vi "PQ-12 quick release (SubVI).vi"(1 "error in (no error)":errorcluster, 2 "output cluster":T26 {"A/SPI - LiDAR"."SPI Configuration"."Frame Length" min=1 max=16}, 3 "Extend / Retract [F/T]":bool) -> (0 "error out":errorcluster)   [LabVIEW 2018]
uses:
  <vilib>/myRIO/Instrument Drivers/Onboard IO/DIO/typedefs/DIO Reference.ctl
  <vilib>/myRIO/Common/Instrument Driver Framework/Utilities/typedefs/myRIO Generic Hardware Reference.ctl
  <vilib>/myRIO/Common/Instrument Driver Framework/Utilities/typedefs/Hardware Version Enum.ctl
  <vilib>/myRIO/Common/Instrument Driver Framework/Utilities/typedefs/myRIO v1.0 Reference.ctl
  <vilib>/myRIO/Common/Instrument Driver Framework/Utilities/typedefs/Generic FPGA Reference.ctl
  <vilib>/myRIO/Common/Instrument Driver Framework/myRIO v1.0/DIO/typedefs/DIO Channels List.ctl
  <vilib>/myRIO/Common/Instrument Driver Framework/myRIO v1.0/DIO/typedefs/DIO Channels Enum.ctl
  <vilib>/myRIO/Instrument Drivers/Onboard IO/PWM/typedefs/PWM Reference.ctl
  <vilib>/myRIO/Common/Instrument Driver Framework/myRIO v1.0/PWM/typedefs/PWM Channels Enum.ctl
  <vilib>/myRIO/Instrument Drivers/Onboard IO/PWM/typedefs/PWM Configuration.ctl
  <vilib>/myRIO/Instrument Drivers/Onboard Devices/Accelerometer/typedefs/Accelerometer Reference.ctl
  <vilib>/myRIO/Common/Instrument Driver Framework/myRIO v1.0/Accelerometer/typedefs/Accelerometer Channels List.ctl
  <vilib>/myRIO/Common/Instrument Driver Framework/myRIO v1.0/Accelerometer/typedefs/Accelerometer Channels Enum.ctl
  <vilib>/myRIO/Instrument Drivers/Onboard IO/AI/typedefs/AI Reference.ctl
  <vilib>/myRIO/Common/Instrument Driver Framework/myRIO v1.0/AI/typedefs/AI Channels List.ctl
  <vilib>/myRIO/Common/Instrument Driver Framework/myRIO v1.0/AI/typedefs/AI Channels Enum.ctl
  <vilib>/myRIO/Common/Instrument Driver Framework/Utilities/typedefs/Analog Scaling Constants List.ctl
  <vilib>/myRIO/Common/Instrument Driver Framework/Utilities/typedefs/Analog Scaling Constants.ctl
  <vilib>/myRIO/Instrument Drivers/Onboard IO/SPI/typedefs/SPI Reference.ctl
  <vilib>/myRIO/Common/Instrument Driver Framework/myRIO v1.0/SPI/typedefs/SPI Channels Enum.ctl
  <vilib>/myRIO/Instrument Drivers/Onboard IO/SPI/typedefs/SPI Configuration.ctl
  <vilib>/myRIO/Common/Instrument Driver Framework/myRIO v1.0/SPI/typedefs/SPI Clock Phase.ctl
  <vilib>/myRIO/Common/Instrument Driver Framework/myRIO v1.0/SPI/typedefs/SPI Clock Polarity.ctl
  <vilib>/myRIO/Common/Instrument Driver Framework/myRIO v1.0/SPI/typedefs/SPI Data Direction.ctl
  <vilib>/myRIO/Common/Instrument Driver Framework/myRIO v1.0/SPI/typedefs/SPI Frame Length.ctl
  <vilib>/Utility/error.llb/Error Cluster From Error Code.vi
  <vilib>/myRIO/Common/Instrument Driver Framework/myRIO v1.0/AI/vis/myRIO v1.0 Read AI.vi
  <vilib>/myRIO/Common/Instrument Driver Framework/myRIO v1.0/DIO/vis/myRIO v1.0 Write DIO.vi
  <vilib>/myRIO/Instrument Drivers/Onboard IO/AI/AI.lvlib
  <vilib>/myRIO/Instrument Drivers/Onboard IO/DIO/DIO.lvlib
  <vilib>/myRIO/Instrument Drivers/Onboard IO/SPI/SPI.lvlib
  <vilib>/myRIO/Instrument Drivers/Onboard Devices/Accelerometer/Accelerometer.lvlib
  <vilib>/myRIO/Instrument Drivers/Onboard IO/PWM/PWM.lvlib
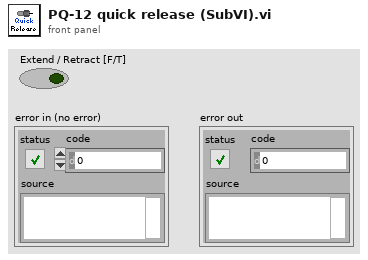
[diagram p1: front panel]
types:
  T1 = typedef "DIO.lvlib/DIO Reference.ctl" = cluster{"myRIO Reference":T2, "DIO Channels List":T6}
  T2 = typedef "myRIO Generic Hardware Reference.ctl" = cluster{"myRIO Model":T3, "myRIO Hardware Reference":T4}
  T3 = typedef "Hardware Version Enum.ctl" = enum16{"Unknown", "myRIO-1900", "myRIO-1950", "roboRIO", "NI ELVIS RIO CM", "ELVIS III"}
  T4 = typedef "myRIO v1.0 Reference.ctl" = cluster{"Generic FPGA Reference":T5, "Allow multiple opens":bool}
  T5 = typedef "Generic FPGA Reference.ctl" = refnum<k20>
  T6 = typedef "DIO Channels List.ctl" = T7[]
  T7 = typedef "DIO Channels Enum.ctl" = enum16{"Not Connected", "C/DIO0", "C/DIO1", "C/DIO2", "C/DIO3", "C/DIO4", "C/DIO5", "C/DIO6", "C/DIO7", "A/DIO0", "A/DIO1", "A/DIO2", "A/DIO3", "A/DIO4", "A/DIO5", "A/DIO6", "A/DIO7", "A/DIO8", "A/DIO9", "A/DIO10", "A/DIO11", "A/DIO12", "A/DIO13", "A/DIO14", "A/DIO15", "A/DIO16", "A/DIO17", "A/DIO18", "A/DIO19", "B/DIO0", "B/DIO1", "B/DIO2", "B/DIO3", "B/DIO4", "B/DIO5", "B/DIO6", "B/DIO7", "B/DIO8", "B/DIO9", "B/DIO10", "B/DIO11", "B/DIO12", "B/DIO13", "B/DIO14", "B/DIO15", "B/DIO16", "B/DIO17", "B/DIO18", "B/DIO19", "LED0", "LED1", "LED2", "LED3", "Button0", "DIO/DIO0", "DIO/DIO1", "DIO/DIO2", "DIO/DIO3", "DIO/DIO4", "DIO/DIO5", "DIO/DIO6", "DIO/DIO7", "DIO/DIO8", "DIO/DIO9", "SPI/CS0", "SPI/CS1", "SPI/CS2", "SPI/CS3", "LED RADIO (Green)", "LED RADIO (Red)", "LED COMM (Green)", "LED COMM (Red)", "LED MODE (Green)", "LED MODE (Red)"}
  T8 = typedef "PWM.lvlib/PWM Reference.ctl" = cluster{"myRIO Reference":T2, "PWM Channels Enum":T9, "PWM Configuration":T10}
  T9 = typedef "PWM Channels Enum.ctl" = enum16{"Not Connected", "C/PWM0", "C/PWM1", "A/PWM0", "A/PWM1", "A/PWM2", "A/PWM3", "A/PWM4", "A/PWM5", "A/PWM6", "A/PWM7", "A/PWM8", "A/PWM9", "A/PWM10", "A/PWM11", "A/PWM12", "A/PWM13", "A/PWM14", "A/PWM15", "A/PWM16", "A/PWM17", "A/PWM18", "A/PWM19", "B/PWM0", "B/PWM1", "B/PWM2", "B/PWM3", "B/PWM4", "B/PWM5", "B/PWM6", "B/PWM7", "B/PWM8", "B/PWM9", "B/PWM10", "B/PWM11", "B/PWM12", "B/PWM13", "B/PWM14", "B/PWM15", "B/PWM16", "B/PWM17", "B/PWM18", "B/PWM19", "PWM/PWM0", "PWM/PWM1", "PWM/PWM2", "PWM/PWM3", "PWM/PWM4", "PWM/PWM5", "PWM/PWM6", "PWM/PWM7", "PWM/PWM8", "PWM/PWM9"}
  T10 = typedef "PWM.lvlib/PWM Configuration.ctl" = cluster{"Frequency":dbl, "Duty Cycle":dbl}
  T11 = typedef "Accelerometer.lvlib/Accelerometer Reference.ctl" = cluster{"myRIO Reference":T2, "Accelerometer Channels List":T12, "LSB Weight":dbl}
  T12 = typedef "Accelerometer Channels List.ctl" = T13[]
  T13 = typedef "Accelerometer Channels Enum.ctl" = enum16{"Not Connected", "X-Axis", "Y-Axis", "Z-Axis"}
  T14 = typedef "AI.lvlib/AI Reference.ctl" = cluster{"myRIO Reference":T2, "AI Channels List":T15, "AI Scaling Constants List":T17}
  T15 = typedef "AI Channels List.ctl" = T16[]
  T16 = typedef "AI Channels Enum.ctl" = enum16{"Not Connected", "AudioIn/Left", "AudioIn/Right", "C/AI0", "C/AI1", "A/AI0", "A/AI1", "A/AI2", "A/AI3", "A/AI4", "A/AI5", "A/AI6", "A/AI7", "B/AI0", "B/AI1", "B/AI2", "B/AI3", "B/AI4", "B/AI5", "B/AI6", "B/AI7", "AI/AI0", "AI/AI1", "AI/AI2", "AI/AI3", "A/AI0 (DIFF)", "A/AI1 (DIFF)", "A/AI2 (DIFF)", "A/AI3 (DIFF)", "B/AI0 (DIFF)", "B/AI1 (DIFF)", "B/AI2 (DIFF)", "B/AI3 (DIFF)"}
  T17 = typedef "Analog Scaling Constants List.ctl" = T18[]
  T18 = typedef "Analog Scaling Constants.ctl" = cluster{"LSB Weight (Volts)":dbl, "Offset (Volts)":dbl, "Signed?":bool}
  T19 = typedef "SPI.lvlib/SPI Reference.ctl" = cluster{"myRIO Reference":T2, "SPI Channels Enum":T20, "SPI Configuration":T21}
  T20 = typedef "SPI Channels Enum.ctl" = enum16{"Not Connected", "A/SPI", "B/SPI", "SPI/SPI"}
  T21 = typedef "SPI.lvlib/SPI Configuration.ctl" = cluster{"Frequency [Hz]":dbl, "Clock Phase":T22, "Clock Polarity":T23, "Data Direction":T24, "Frame Length":T25}
  T22 = typedef "SPI Clock Phase.ctl" = enum8{"Leading", "Trailing"}
  T23 = typedef "SPI Clock Polarity.ctl" = enum8{"Low", "High"}
  T24 = typedef "SPI Data Direction.ctl" = enum8{"Most significant bit first", "Least significant bit first"}
  T25 = typedef "SPI Frame Length.ctl" = u8
  T26 = cluster{"B/DIO0 - Stepper Direction":T1, "B/DIO1 - Stepper1 Enable":T1, "B/DIO2 - Stepper2 Enable":T1, "B/DIO3 - Stepper3 Enable":T1, "B/DIO4 - Endstop Stepper1 Top":T1, "B/DIO11 - Endstop Stepper1 Bund":T1, "B/DIO12 - Endstop Stepper2 Top":T1, "B/DIO13 - Endstop Stepper2 Bund":T1, "B/DIO14 - Endstop Stepper3 Top":T1, "B/DIO15 - Endstop Stepper3 Bund":T1, "A/DIO0 - Cooler":T1, "A/DIO1 - Beacon drop (dio1)":T1, "A/DIO2 - Beacon drop (dio0)":T1, "A/DIO3 - QuickRelease (dio1)":T1, "A/DIO4 - QuickRelease (dio0)":T1, "A/DIO11 - LiDAR SPI CS":T1, "B/PWM0 - Stepper":T8, "B/PWM1 - Drill":T8, "A/PWM0 - Servo_Roll":T8, "A/PWM1 - Servo_Yaw":T8, "Acc. X-axis":T11, "Acc. Y-axis":T11, "B/AI0 - Drone Grounded F3":T14, "B/AI1 - Drone Drill Gear F4":T14, "B/AI2 - Beacon Drop F5":T14, "B/AI3 - Drone Drill Boost F6":T14, "A/AI0 - Drone Stepper F8":T14, "A/AI1 - Beacon Wiper":T14, "A/AI2 - QuickRelease Wiper":T14, "A/AI3 - Drill Current":T14, "A/SPI - LiDAR":T19, "B/UART - XBee":refnum<visa-resource-name>, "A/UART - A3 GPS":refnum<visa-resource-name>, "RIO Flashing LEDs":T1}
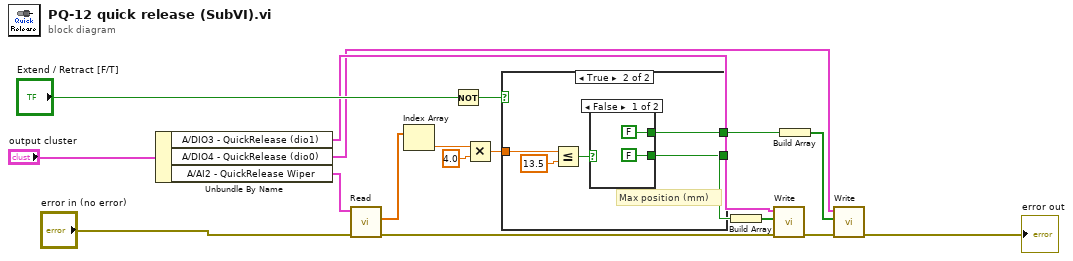
[diagram p0: block diagram]
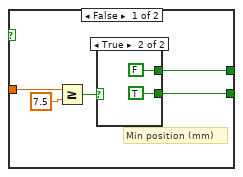
[diagram p2: hidden frame]
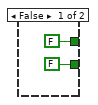
[diagram p3: hidden frame]
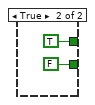
[diagram p4: hidden frame]
diagram:
  n1 = Unbundle By Name("output cluster") -> ("A/DIO3 - QuickRelease (dio1)"=w3:T1, "A/DIO4 - QuickRelease (dio0)"=w2:T1, "A/AI2 - QuickRelease Wiper"=w4:T14)
  n2 = call <vilib>:"Read.vi"("error in (no error)"="error in (no error)", "AI Ref In"=w4) -> ("error out"=w7:errorcluster, "Values"=w17:dbl[])  [unwired: 7 in, 1 out]
  n3 = Index Array(array=w17) -> (element=w18:dbl)  [unwired: 1 in]
  n4 = Not(x="Extend / Retract [F/T]") -> (.not. x?=w11:bool)
  n5 = Multiply(x=w18, y=4.0) -> (x*y=w16:dbl)
  n6 = case shown="True" w11 {
    tunnel: [w23 w32] -> w14
    tunnel: [w22 w31] -> w6
    tunnel: w16 -> [w20 w29]
    frame False {
      # "Min position (mm)"
      n7 = Greater Or Equal?(x=w20, y=7.5) -> (x >= y?=w21:bool)
      n8 = case shown="True" w21 {
        tunnel: [FALSE FALSE] -> w23
        tunnel: [FALSE TRUE] -> w22
        frame False {
        }
        frame True {
        }
      }
    }
    frame True {
      # "Max position (mm)"
      n9 = Less Or Equal?(x=w29, y=13.5) -> (x <= y?=w30:bool)
      n10 = case shown="False" w30 {
        tunnel: [FALSE TRUE] -> w32
        tunnel: [FALSE FALSE] -> w31
        frame False {
        }
        frame True {
        }
      }
    }
  }
  n11 = Build Array(w6) -> (w5:bool[])
  n12 = call <vilib>:"Write.vi"("error in (no error)"=w7, "Values"=w5, "DIO Ref In"=w3) -> ("error out"=w8:errorcluster)  [unwired: 6 in, 1 out]
  n13 = Build Array(w14) -> (w13:bool[])
  n14 = call <vilib>:"Write.vi"("error in (no error)"=w8, "Values"=w13, "DIO Ref In"=w2) -> ("error out"=→"error out":errorcluster)  [unwired: 6 in, 1 out]
